vi "Call.vi"(7 "Actor in":refnum<class "Actor.lvclass">, 10 "Msg":refnum<class "Msg.lvclass">) -> (0 "Error out":errorcluster, 2 "Msg Output":refnum<class "Msg Output.lvclass">, 5 "Actor out":refnum<class "Actor.lvclass">)   [LabVIEW 2025, in "jettl.lvlib"]
uses:
  jettl.lvlib
  Actor/Actor.lvclass
  Msg/Msg.lvclass
  Msg Output/Msg Output.lvclass
  Attributes/Attributes/Attributes.lvclass
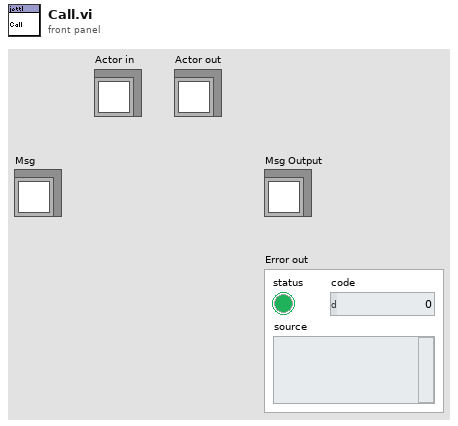
[diagram p1: front panel]
types:
  T1 = typedef "jettl.lvlib/Msg Set.ctl" = set{refnum<class "Msg.lvclass">}
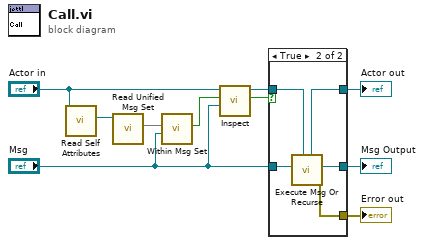
[diagram p0: block diagram]
diagram:
  n1 = call-dynamic "Read Self Attributes.vi"("Actor in"="Actor in") -> ("Self Attributes"=w10:refnum<class "Attributes.lvclass">)  [unwired: 10 in]
  n2 = call-dynamic "Read Unified Msg Set.vi"("Attributes in"=w10) -> ("Unified Msg Set"=w9:T1)  [unwired: 10 in]
  n3 = call "Within Msg Set.vi"("Msg"="Msg", "Msg Set"=w9) -> ("Within Msg Set"=w8:bool)  [unwired: 9 in]
  n4 = call-dynamic "Inspect.vi"("Msg in"="Msg", "Within Msg Set"=w8, "Actor in"="Actor in") -> ("Execute Msg Or Recurse"=w1:bool, "Actor out"=w4:refnum<class "Actor.lvclass">)  [unwired: 7 in]
  n5 = case shown="True" w1 {
    tunnel: w4 -> [w11 w16]
    tunnel: [w11 w15] -> w6
    tunnel: "Msg" -> [_ w13]
    tunnel: [_ w14] -> w5
    tunnel: [_ w12] -> w3
    frame False {
    }
    frame True {
      n6 = call "Execute Msg Or Recurse.vi"("Actor in"=w16, "Msg"=w13) -> ("Error out"=w14:errorcluster, "Msg Output"=w12:refnum<class "Msg Output.lvclass">, "Actor out"=w15:refnum<class "Actor.lvclass">)  [unwired: 7 in]
    }
  }
  "Actor out" <- w6
  "Error out" <- w5
  "Msg Output" <- w3
